vi "sv_Convert FRF Results.vi"(0 "magnitudes":cluster{"X":dbl[], "Y":dbl[]}[](array[cluster]) {"X" format="%.2f"; "Y" format="%.2f"}, 1 "ref amplitude":dbl, 5 "Phases":cluster{"X":dbl[], "Y":dbl[]}[](array[cluster]) {"X" format="%.2f"; "Y" format="%.2f"}, 7 "reference channel":i32=-1, 12 "view":T1={"dB On? (T)"=TRUE, "unwrap phase? (F)"=FALSE, "convert to degree? (T)"=TRUE}) -> (3 "Units":cluster{string, string}[](array[cluster]), 4 "Magnitudes":cluster{"X":dbl[], "Y":dbl[]}[](array[cluster]), 6 "Phases":cluster{"X":dbl[], "Y":dbl[]}[](array[cluster]))   [LabVIEW 2017, in "SoundVib_ContSweptSine.lvlib"]
uses:
  <vilib>/addons/Sound and Vibration/svt_Continuous Swept Sine/SoundVib_ContSweptSine.lvlib
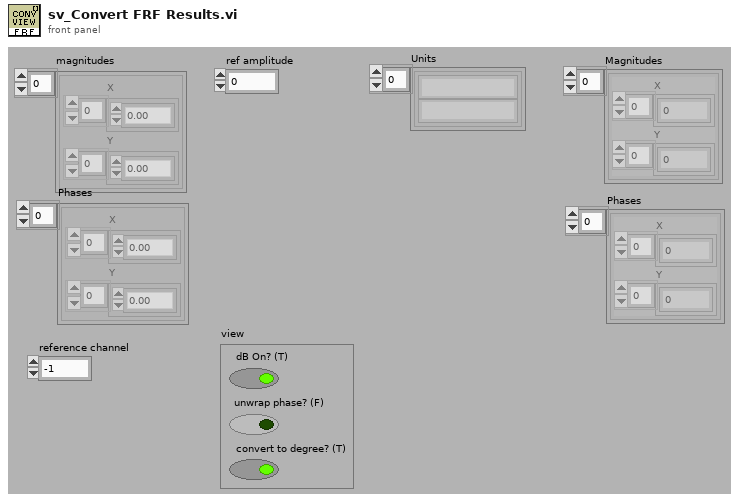
[diagram p1: front panel]
types:
  T1 = cluster{"dB On? (T)":bool, "unwrap phase? (F)":bool, "convert to degree? (T)":bool}
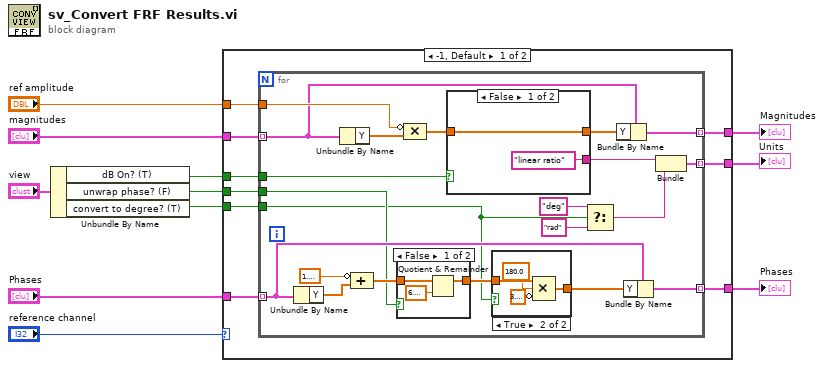
[diagram p0: block diagram]
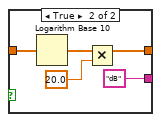
[diagram p2: hidden frame]
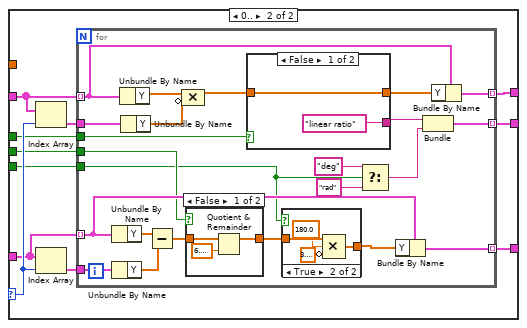
[diagram p5: hidden frame]
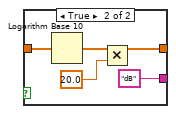
[diagram p6: hidden frame]
diagram:
  n1 = Unbundle By Name("view") -> ("dB On? (T)"=w6:bool, "unwrap phase? (F)"=w5:bool, "convert to degree? (T)"=w4:bool)
  n2 = case shown="-1, Default" "reference channel" {
    selector: "reference channel" -> [_ w64]
    tunnel: "magnitudes" -> [w20 w67]
    tunnel: [w19 w68] -> w3
    tunnel: "ref amplitude" -> [w18 _]
    tunnel: [w17 w65] -> w2
    tunnel: "Phases" -> [w16 w62]
    tunnel: [w15 w61] -> w1
    tunnel: w6 -> [w14 w60]
    tunnel: w5 -> [w13 w59]
    tunnel: w4 -> [w12 w58]
    frame -1, Default {
      n3 = for {
        tunnel: w20 -> [w39] mode=indexing
        tunnel: w18 -> [w40]
        tunnel: [w37] -> w19 mode=indexing
        tunnel: [w38] -> w17 mode=indexing
        tunnel: w16 -> [w34] mode=indexing
        tunnel: [w32] -> w15 mode=indexing
        tunnel: w14 -> [w27]
        tunnel: w13 -> [w26]
        tunnel: w12 -> [w24]
        n4 = Unbundle By Name(w34) -> ("Y"=w35:dbl[])
        n5 = Unbundle By Name(w39) -> ("Y"=w41:dbl[])
        n6 = Compound Arithmetic op=ADD(invert 1.5707963267948966, w35) -> (w31:dbl[])
        n7 = case shown="False" w26 {
          tunnel: w31 -> [w54 w57]
          tunnel: [w55 w57] -> w36
          frame False {
            n8 = Quotient & Remainder(x=w54, y=6.283185307179586) -> (x-y*floor(x/y)=w55:dbl[])  [unwired: 1 out]
          }
          frame True {
          }
        }
        n9 = Compound Arithmetic op=MULTIPLY(invert w40, w41) -> (w29:dbl[])
        n10 = case shown="False" w27 {
          tunnel: [w43 w45] -> w28
          tunnel: w29 -> [w43 w48]
          tunnel: ["linear ratio" "dB"] -> w25
          frame False {
          }
          frame True {
            n11 = Logarithm Base 10(1:w48) -> (0:w47:dbl[])
            n12 = Multiply(x=w47, y=20.0) -> (x*y=w45:dbl[])
          }
        }
        n13 = case shown="True" w24 {
          tunnel: w36 -> [w49 w53]
          tunnel: [w49 w52] -> w33
          frame False {
          }
          frame True {
            n14 = Compound Arithmetic op=MULTIPLY(w53, 180.0, invert 3.141592653589793) -> (w52:dbl[])
          }
        }
        n15 = Select(t="deg", s=w24, f="rad") -> (s? t:f=w21:string)
        n16 = Bundle By Name(cluster=w39, "Y"=w28) -> (w37:cluster{"X":dbl[], "Y":dbl[]})
        n17 = Bundle By Name(cluster=w34, "Y"=w33) -> (w32:cluster{"X":dbl[], "Y":dbl[]})
        n18 = Bundle(w25, w21) -> (w38:cluster{string, string})  [unwired: 1 in]
      }
    }
    frame 0.. {
      n19 = Index Array(array=w67, index=w64) -> (element=w66:cluster{"X":dbl[], "Y":dbl[]})
      n20 = Index Array(array=w62, index=w64) -> (element=w63:cluster{"X":dbl[], "Y":dbl[]})
      n21 = for {
        tunnel: w67 -> [w88] mode=indexing
        tunnel: [w86] -> w68 mode=indexing
        tunnel: w66 -> [w90]
        tunnel: [w87] -> w65 mode=indexing
        tunnel: w63 -> [w85]
        tunnel: w62 -> [w80] mode=indexing
        tunnel: [w78] -> w61 mode=indexing
        tunnel: w60 -> [w74]
        tunnel: w59 -> [w73]
        tunnel: w58 -> [w70]
        n22 = Unbundle By Name(w80) -> ("Y"=w84:dbl[])
        n23 = Unbundle By Name(w85) -> ("Y"=w83:dbl[])
        n24 = Unbundle By Name(w88) -> ("Y"=w91:dbl[])
        n25 = Unbundle By Name(w90) -> ("Y"=w89:dbl[])
        n26 = Subtract(x=w84, y=w83) -> (x-y=w82:dbl[])
        n27 = Compound Arithmetic op=MULTIPLY(w91, invert w89) -> (w77:dbl[])
        n28 = case shown="False" w73 {
          tunnel: w82 -> [w106 w107]
          tunnel: [w104 w107] -> w81
          frame False {
            n29 = Quotient & Remainder(x=w106, y=6.283185307179586) -> (x-y*floor(x/y)=w104:dbl[])  [unwired: 1 out]
          }
          frame True {
          }
        }
        n30 = case shown="False" w74 {
          tunnel: [w93 w95] -> w76
          tunnel: w77 -> [w93 w98]
          tunnel: ["linear ratio" "dB"] -> w75
          frame False {
          }
          frame True {
            n31 = Logarithm Base 10(1:w98) -> (0:w97:dbl[])
            n32 = Multiply(x=w97, y=20.0) -> (x*y=w95:dbl[])
          }
        }
        n33 = case shown="True" w70 {
          tunnel: w81 -> [w99 w103]
          tunnel: [w99 w102] -> w79
          frame False {
          }
          frame True {
            n34 = Compound Arithmetic op=MULTIPLY(w103, 180.0, invert 3.141592653589793) -> (w102:dbl[])
          }
        }
        n35 = Select(t="deg", s=w70, f="rad") -> (s? t:f=w69:string)
        n36 = Bundle By Name(cluster=w80, "Y"=w79) -> (w78:cluster{"X":dbl[], "Y":dbl[]})
        n37 = Bundle(w75, w69) -> (w87:cluster{string, string})  [unwired: 1 in]
        n38 = Bundle By Name(cluster=w88, "Y"=w76) -> (w86:cluster{"X":dbl[], "Y":dbl[]})
      }
    }
  }
  "Magnitudes" <- w3
  "Units" <- w2
  "Phases" <- w1
